vi "Analysis.GUI.vi"(11 "Parameters":T1={"Results Path"=path "C:/testdata/Logs", "Temp Path"=path "C:/testdata/Temp", "Remote Path"=path "d:/testdata/Logs", "Analysis VIs"=[path "C:/addons/TestStand Examples for HIL/Continuous Monitoring Tester/Sequences/Analysis/Builds/TestStand Analysis Steps.lvlibp/Post Process Analysis Steps/Analysis.LevelTransition.vi"], "Report Passed?"=FALSE, "Group Channels?"=FALSE}) -> ()   [LabVIEW 2015, in "Analysis.lvlib"]
uses:
  Analysis.lvlib
  Types/Analysis.GUI.Parameters.ctl
  Types/Analysis.GUI.Refs.ctl
panel:
  out "Cycle":i32
  in  "error in (no error)":errorcluster
  out "Results Directory":path=path "d:/testdata/TestResults"
  in  "Results":string(tree)
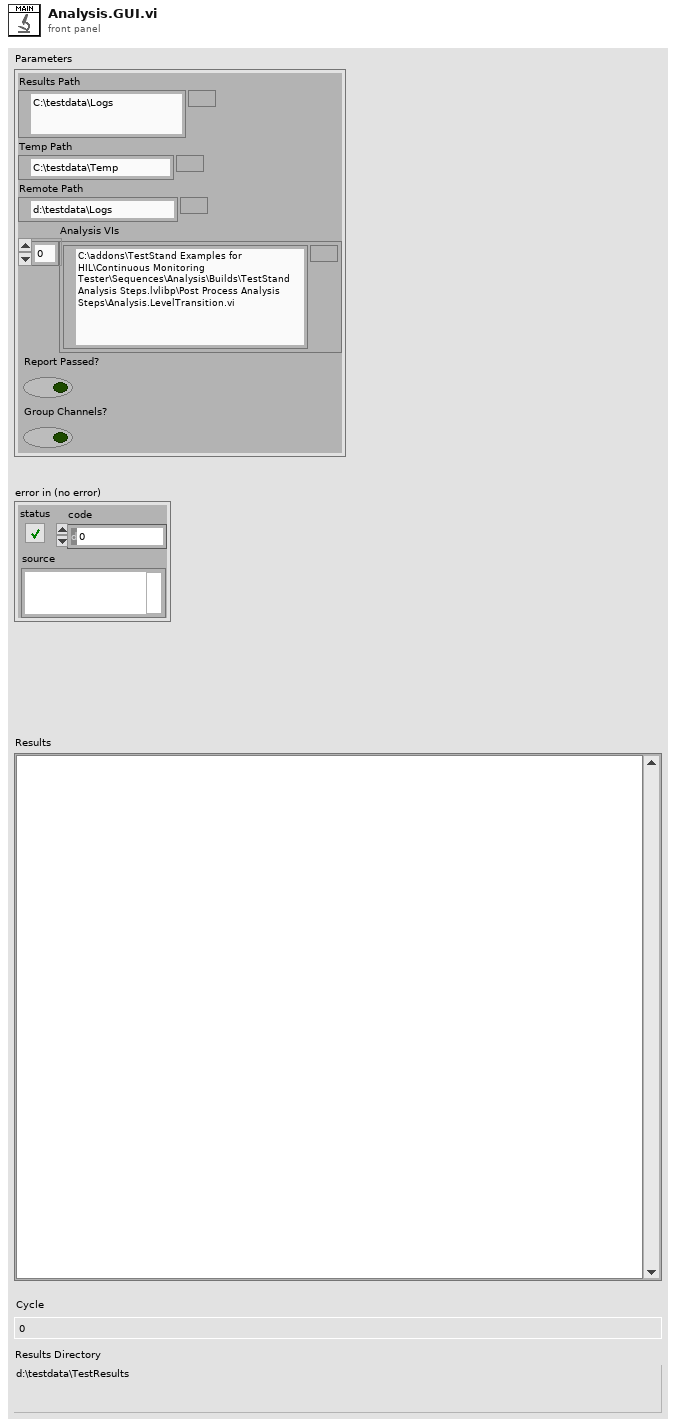
[diagram p1: front panel]
types:
  T1 = typedef "Analysis.lvlib/Analysis.GUI.Parameters.ctl" = cluster{"Results Path":path, "Temp Path":path, "Remote Path":path, "Analysis VIs":path[], "Report Passed?":bool, "Group Channels?":bool}
  T2 = typedef "Analysis.lvlib/Analysis.GUI.Refs.ctl" = cluster{"Cycle":refnum<vi>, "Tree":refnum<vi>, " VI":refnum<vi>, "Results.Directory":refnum<vi>}
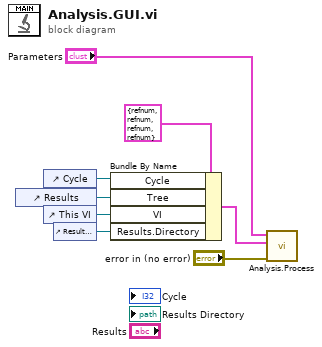
[diagram p0: block diagram]
diagram:
  n1 = control-ref of="Results"() -> (w7:refnum<vi>)
  n2 = control-ref of="Cycle"() -> (w5:refnum<vi>)
  n3 = control-ref of="This VI"() -> (w4:refnum<vi>)
  n4 = control-ref of="Results Directory"() -> (w3:refnum<vi>)
  n5 = Bundle By Name(cluster=T2 {"Cycle"=refnum, "Tree"=refnum, " VI"=refnum, "Results.Directory"=refnum} ("output cluster"), "Cycle"=w5, "Tree"=w7, "VI"=w4, "Results.Directory"=w3) -> (w1:T2)
  n6 = call "Analysis.Process.vi"("error in (no error)"="error in (no error)", "Refs"=w1, "Parameters"="Parameters") -> ()  [unwired: 9 in]
